vi "NI9219_InputConfig.vi"(8 "Stop":bool, 9 "Number of Samples":i32=1000, 10 "Sample Rate":dbl=1000.0 format="%0.2f", 11 "Voltage Input Channels":tag) -> (3 "data":waveform(dbl)[](array[waveform]))   [LabVIEW 2022 SP3]
uses:
  <vilib>/Utility/error.llb/DialogType.ctl
  <vilib>/DAQmx/read.llb/DAQmx Read (Analog 1D Wfm NChan NSamp).vi
  <vilib>/DAQmx/create/channels.llb/DAQmx Create Channel (AI-Voltage-Basic).vi
  <vilib>/DAQmx/configure/timing.llb/DAQmx Timing (Sample Clock).vi
  <vilib>/DAQmx/miscellaneous.llb/DAQmx Fill In Error Info.vi
  <resource>/objmgr/daqmx.rc
panel:
  out "Chart for Multiple Channels":waveform(dbl)[](graph)
  out "Graph for Multiple Channels":waveform(dbl)[](graph)
  out "SampClk.Rate":dbl
  # "Voltage Input NI 9219"
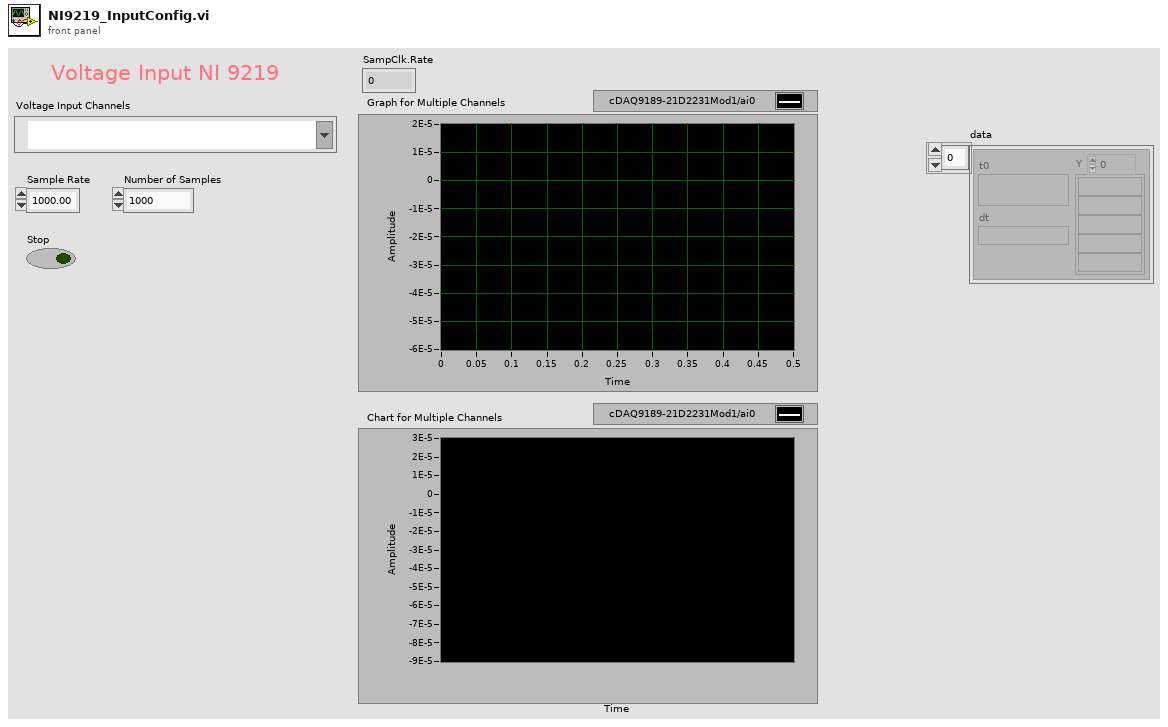
[diagram p1: front panel]
types:
  T1 = typedef "DialogType.ctl" = u16
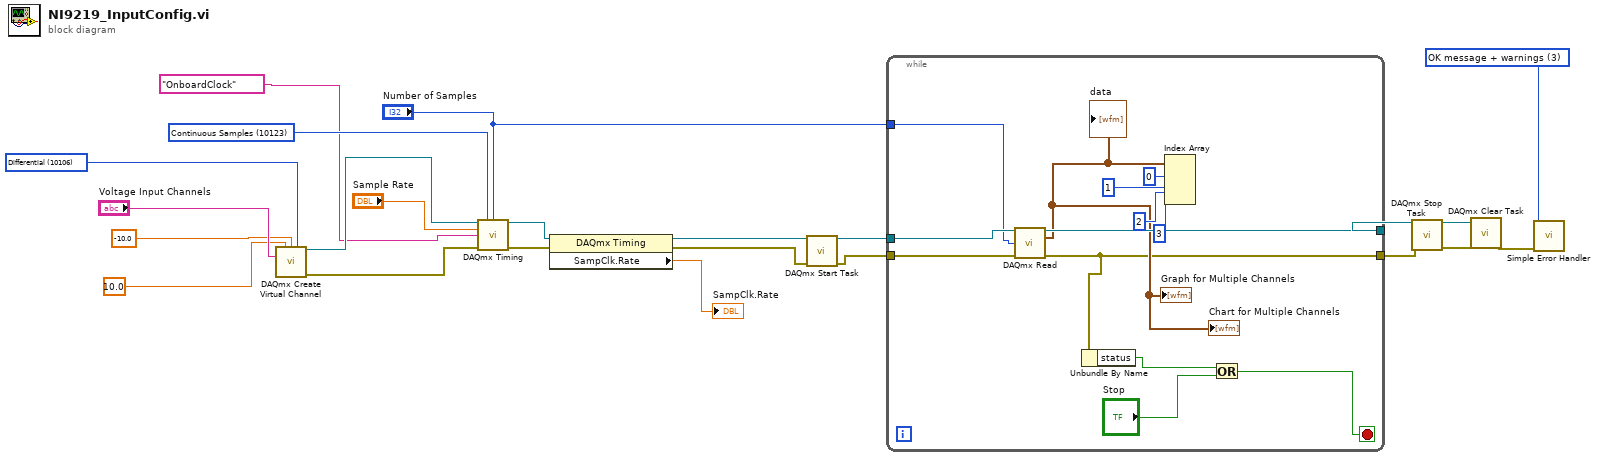
[diagram p0: block diagram]
diagram:
  w1 = T1 3 items=["no dialog", "OK message", "continue or stop message", "OK message + warnings", "continue/stop + warnings"] ("type of dialog (OK msg:1)")
  w13 = 10123 items=["Finite Samples"=10178, "Continuous Samples"=10123, "Hardware Timed Single Point"=12522] ("sample mode")
  w20 = 10106 items=["Default"=-1, "RSE"=10083, "NRSE"=10078, "Differential"=10106, "Pseudodifferential"=12529] ("input terminal configuration")
  n1 = call-poly <vilib>:"DAQmx Create Virtual Channel.vi"("maximum value"=10.0, "minimum value"=-10.0, "input terminal configuration"=w20, "physical channels"="Voltage Input Channels") -> ("task out"=w23:refnum<k21>, "error out"=w22:errorcluster)  [unwired: 10 in]
  n2 = call-poly <vilib>:"DAQmx Timing.vi"("task/channels in"=w23, "sample mode"=w13, "samples per channel"="Number of Samples", "rate"="Sample Rate", "source"=tag "OnboardClock", "error in"=w22) -> ("task out"=w18:refnum<k21>, "error out"=w17:errorcluster)  [unwired: 8 in]
  n3 = property class="DAQmx Timing"(reference=w18, error in=w17) -> (reference out=w10:refnum<k21>, error out=w11:errorcluster, "SampClk.Rate"=→"SampClk.Rate":dbl)
  n4 = call <vilib>:"DAQmx Start Task.vi"("task/channels in"=w10, "error in"=w11) -> ("task out"=w9:refnum<k21>, "error out"=w8:errorcluster)  [unwired: 12 in]
  n5 = while {
    tunnel: w9 -> [w36]
    tunnel: w8 -> [w35]
    tunnel: "Number of Samples" -> [w34]
    tunnel: [w33] -> w6
    tunnel: [w27] -> w5
    stop <- w24 stop-if-true
    n6 = call-poly <vilib>:"DAQmx Read.vi"("task/channels in"=w36, "number of samples per channel"=w34, "error in"=w35) -> ("task out"=w33:refnum<k21>, "data"=w29:waveform(dbl)[], "error out"=w27:errorcluster)  [unwired: 10 in]
    "Graph for Multiple Channels" <- w29
    "Chart for Multiple Channels" <- w29
    "data" <- w29
    n7 = Unbundle By Name(w27) -> ("status"=w25:bool)
    n8 = Index Array(array=w29, index #1=0 ("index"), index #2=1 ("index"), index #3=2 ("index"), index #4=3 ("index")) -> ()  [unwired: 4 out]
    n9 = Or(x=w25, y="Stop") -> (x .or. y?=w24:bool)
  }
  n10 = call <vilib>:"DAQmx Stop Task.vi"("task/channels in"=w6, "error in"=w5) -> ("task out"=w3:refnum<k21>, "error out"=w4:errorcluster)  [unwired: 12 in]
  n11 = call <vilib>:"DAQmx Clear Task.vi"("task in"=w3, "error in"=w4) -> ("error out"=w2:errorcluster)  [unwired: 13 in]
  n12 = call <vilib>:"Simple Error Handler.vi"("type of dialog (OK msg:1)"=w1, "error in (no error)"=w2) -> ()  [unwired: 3 in, 5 out]
